vi "CalVal-Create Stimulus.vi"(0 "Params":T1, 7 "Test Freq (Hz)":dbl, 11 "error in (no error)":errorcluster) -> (15 "error out":errorcluster)   [LabVIEW 2020]
uses:
  Type Defs/CalVal-Params.ctl
  Utility VIs/Type Defs/Left-Right ring.ctl
  PXI DAQ VIs/DAQ Engine VIs/PXI Globals.vi
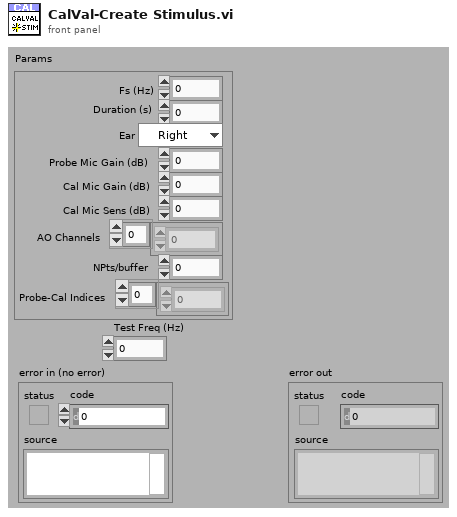
[diagram p1: front panel]
types:
  T1 = typedef "CalVal-Params.ctl" = cluster{"Fs (Hz)":dbl, "Duration (s)":dbl, "Ear":T2, "Probe Mic Gain (dB)":dbl, "Cal Mic Gain (dB)":dbl, "Cal Mic Sens (dB)":dbl, "AO Channels":i32[], "NPts/buffer":i32, "Probe-Cal Indices":i32[]}
  T2 = typedef "Left-Right ring.ctl" = enum16{"Right", "Left"}
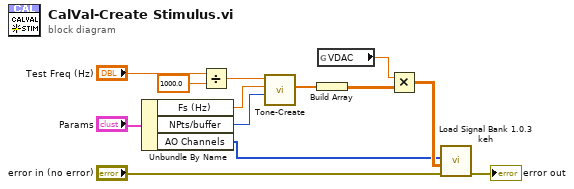
[diagram p0: block diagram]
diagram:
  n1 = Unbundle By Name("Params") -> ("Fs (Hz)"=w4:dbl, "NPts/buffer"=w5:i32, "AO Channels"=w6:i32[])
  n2 = Divide(x="Test Freq (Hz)", y=1000.0) -> (x/y=w2:dbl)
  n3 = call "Tone-Create.vi"("Npts"=w5, "Sampling Rate (Hz)"=w4, "Frequency (kHz)"=w2) -> ("Waveform"=w12:dbl[])  [unwired: 7 in, 1 out]
  n4 = Build Array(w12) -> (w9:dbl[][])
  n5 = global read "PXI Globals.vi" "VDAC"() -> (w10:dbl)
  n6 = Multiply(x=w10, y=w9) -> (x*y=w11:dbl[][])
  n7 = call "Load Signal Bank 1.0.3 keh.vi"("error in (no error)"="error in (no error)", "Input array"=w11, "Active AO Array"=w6) -> ("error out"=→"error out":errorcluster)  [unwired: 6 in, 2 out]
